vi "3.4.3.vi"() -> ()   [LabVIEW 2018]
panel:
  out "추가된 배열 3":string[](array[string])
  out "추가된 배열 2":string[][](array[string])
  out "추가된 배열":string[](array[string])
  in  "스칼라":string
  in  "배열 2":string[](array[string])
  in  "배열":string[](array[string])
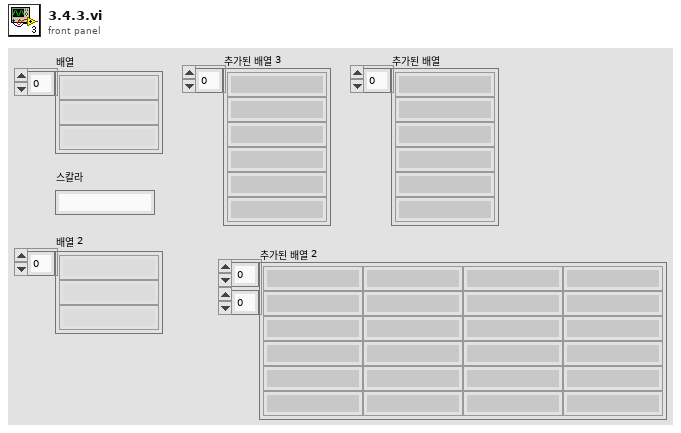
[diagram p1: front panel]
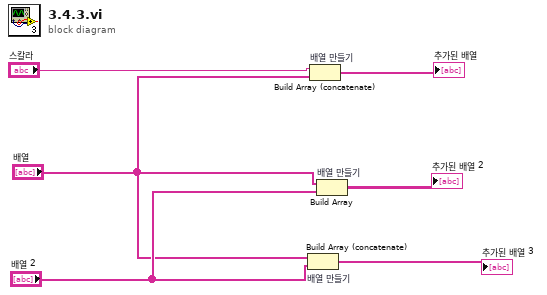
[diagram p0: block diagram]
diagram:
  n1 = Build Array (concatenate) "배열 만들기"("배열", "배열 2") -> (→"추가된 배열 3":string[])
  n2 = Build Array (concatenate) "배열 만들기"("스칼라", "배열") -> (→"추가된 배열":string[])
  n3 = Build Array "배열 만들기"("배열", "배열 2") -> (→"추가된 배열 2":string[][])
